vi "intGreater.vi"(8 "Error in (no error)":errorcluster, 10 "Int2 in":refnum<class "IntClass.lvclass">, 11 "Int1 in":refnum<class "IntClass.lvclass">) -> (0 "Error out":errorcluster, 1 "Timing":u32, 3 "Int1 > Int2?":bool)   [LabVIEW 2011, in "IntClass.lvclass"]
uses:
  IntClass.lvclass
  IntClass.lvclass/IntClass.ctl
  UintClass/UintClass.lvclass
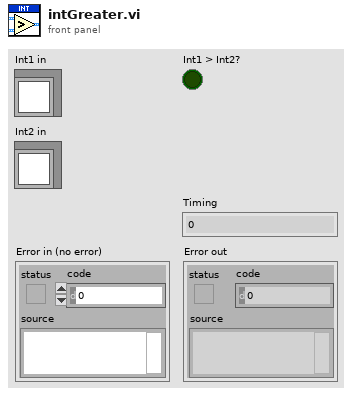
[diagram p1: front panel]
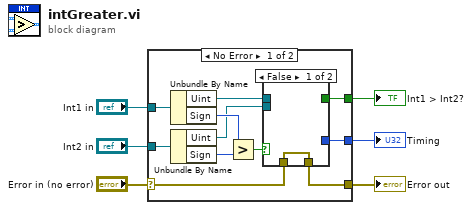
[diagram p0: block diagram]
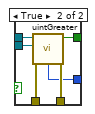
[diagram p2: hidden frame]
diagram:
  n1 = case shown="No Error" "Error in (no error)" {
    selector: "Error in (no error)" -> [w15 w25]
    tunnel: "Int2 in" -> [w16 _]
    tunnel: "Int1 in" -> [w17 _]
    tunnel: [w14 w25] -> w3
    tunnel: [w8 _] -> w2
    tunnel: [w7 _] -> w1
    frame No Error {
      n2 = Unbundle By Name(w17) -> ("Uint"=w11:refnum<class "UintClass.lvclass">, "Sign"=w13:i8)
      n3 = Unbundle By Name(w16) -> ("Uint"=w10:refnum<class "UintClass.lvclass">, "Sign"=w12:i8)
      n4 = Greater?(x=w13, y=w12) -> (0:w9:bool)
      n5 = case shown="False" w9 {
        tunnel: w11 -> [_ w24]
        tunnel: w10 -> [_ w23]
        tunnel: w15 -> [w18 w22]
        tunnel: [w18 w21] -> w14
        tunnel: [_ w20] -> w8
        tunnel: [_ w19] -> w7
        frame False {
        }
        frame True {
          n6 = call "uintGreater.vi"("Error in (no error)"=w22, "Int2 in"=w23, "Int1 in"=w24) -> ("Error out"=w21:errorcluster, "Timing"=w19:u32, "Int1 > Int2?"=w20:bool)  [unwired: 6 in]
        }
      }
    }
    frame Error {
    }
  }
  "Error out" <- w3
  "Timing" <- w1
  "Int1 > Int2?" <- w2
